vi "LDA+_An_Analysis_mode.vi"(6 "Second Graph":T2={"Plot 1"=1, "Plot 2"=2, "Save graph"=0, "Plot Type"=enum."Voltage trace"} {"Save graph" items=["Do not save plot", "Save plot"]; "Plot 2" items=["Nothing", "Prop 2 (U)"]; "Plot 1" items=["Nothing", "Prop 2 (U)"]}, 7 "Running Code?":bool, 9 "First Graph":T2={"Plot 1"=1, "Plot 2"=2, "Save graph"=0, "Plot Type"=enum."Voltage trace"} {"Save graph" items=["Do not save plot", "Save plot"]; "Plot 2" items=["Nothing", "Prop 2 (U)"]; "Plot 1" items=["Nothing", "Prop 2 (U)"]}) -> (0 "Second Graph out":T2={"Plot 1"=1, "Plot 2"=2, "Save graph"=0, "Plot Type"=enum."Voltage trace"} {"Save graph" items=["Do not save plot", "Save plot"]; "Plot 2" items=["Nothing", "Prop 2 (U)"]; "Plot 1" items=["Nothing", "Prop 2 (U)"]}, 3 "First Graph out":T2={"Plot 1"=1, "Plot 2"=2, "Save graph"=0, "Plot Type"=enum."Voltage trace"} {"Save graph" items=["Do not save plot", "Save plot"]; "Plot 2" items=["Nothing", "Prop 2 (U)"]; "Plot 1" items=["Nothing", "Prop 2 (U)"]})   [LabVIEW 2017]
uses:
  Controls/Graph_Type.ctl
  Globals/Meas_global.vi
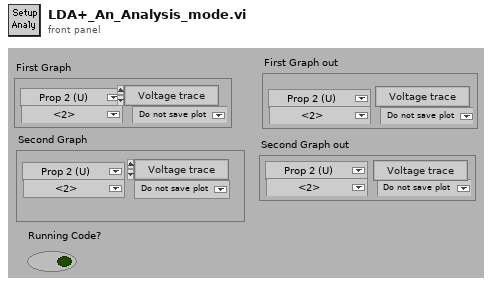
[diagram p1: front panel]
types:
  T1 = typedef "Graph_Type.ctl" = enum16{"Show no graph", "Voltage trace", "Velocity trace", "Vel histogram", "Spectrum", "f.E(f) v Log f", "Auto-Corr"}
  T2 = cluster{"Plot 1":u16, "Plot 2":u16, "Save graph":u16, "Plot Type":T1}
  T3 = typedef "Analysis_info_cluster.ctl" = cluster{"Colour":u32, "Inst type":T4, "Inst name":string, "Symbol":string, "Code name":string, "Extra Info":string, "Inst Array":T5, "Extra Titles":string[], "Extra Values":string[], "U":dbl, "u^2":dbl, "u^3":dbl, "u^4":dbl, "Skew_u":dbl, "Kurt_u":dbl, "Sd Error in Mean":dbl, "% u'/U":dbl, "X":dbl, "Y":dbl, "Z":dbl, "Timescale integral Estimate":dbl, "Sd Error in Variance":dbl, "Calib File":path, "Calib Constants":dbl[], "Output Position":bool, "Full Stats":bool, "Av Sampling Rate":dbl, "Av No of Samples":dbl, "Total Meas Time (s)":dbl, "ADAM Ch Name":string, "Max value":dbl, "Min value":dbl, "Req Sample Rate Hz":dbl, "Sync Delay Time (s)":dbl, "Ch No":i16, "Device ID":string, "Use Latest Calib":bool, "Port":string}
  T4 = typedef "Inst_type.ctl" = enum16{"Propeller anemometer", "Raw voltage", "Pressure Transducer", "Pitot-static tube", "Preston tube", "Hot wire", "Cross wire 1", "Cross wire 2", "Generic Linear", "Generic Polynomial", "Generic BackPoly", "Fast FID", "Thermocouple", "Cold wire", "Pulsed Wire", "LDA Vel", "LDA Tran time", "LDA Arr time", "Microphone"}
  T5 = typedef "Instrument_Array.ctl" = enum16{"PWA", "LDA", "Analogue"}
  T6 = enum16{"Show no graph", "Voltage trace", "Velocity trace", " Vel histogram", "Spectrum", "f.E(f) v Log f", "Auto-Corr"}
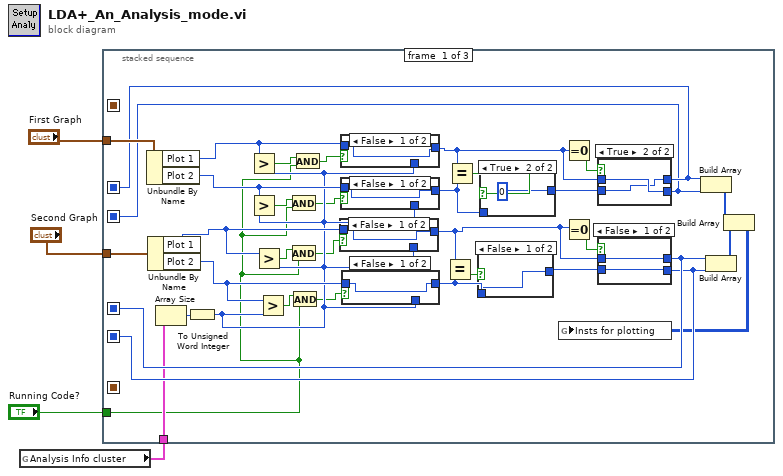
[diagram p0: block diagram]
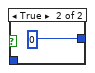
[diagram p9: hidden frame]
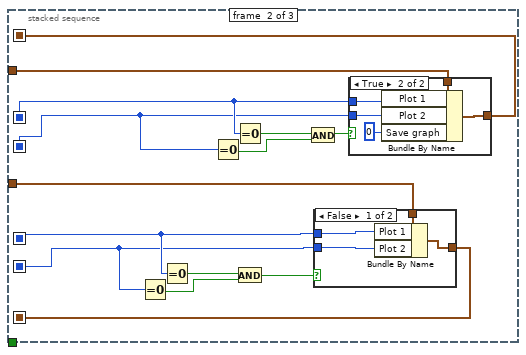
[diagram p10: hidden frame]
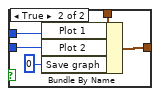
[diagram p11: hidden frame]
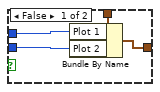
[diagram p12: hidden frame]
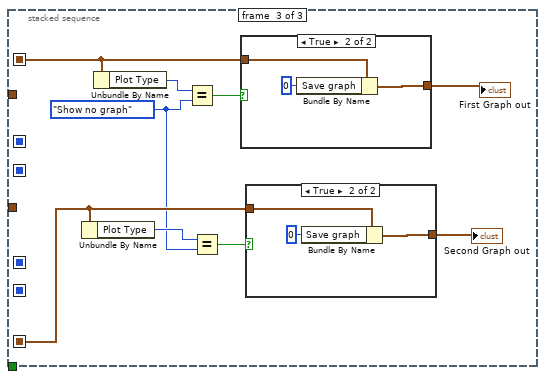
[diagram p13: hidden frame]
diagram:
  n1 = global read "Meas_global.vi" "Analysis Info cluster"() -> (w2:T3[])
  n2 = stacked-sequence {
    seq-local: [w25 _ _] -> [_ w70 _]
    seq-local: [w24 _ _] -> [_ w69 _]
    seq-local: [w20 _ _] -> [_ w64 _]
    seq-local: [w19 _ _] -> [_ w63 _]
    seq-local: [_ w60 _] -> [_ _ w98]
    seq-local: [_ w61 _] -> [_ _ w94]
    tunnel: "First Graph" -> [w34 w73 _]
    tunnel: "Second Graph" -> [w33 w67 _]
    tunnel: w2 -> [w14 _ _]
    tunnel: "Running Code?" -> [w6 _ _]
    frame #0 {
      n3 = Unbundle By Name(w34) -> ("Plot 1"=w32:u16, "Plot 2"=w31:u16)
      n4 = Unbundle By Name(w33) -> ("Plot 1"=w30:u16, "Plot 2"=w29:u16)
      n5 = Array Size(array=w14) -> (size(s)=w39:i32)
      n6 = To Unsigned Word Integer(number=w39) -> (unsigned 16bit integer=w15:u16)
      n7 = Greater?(x=w32, y=w15) -> (0:w12:bool)
      n8 = Greater?(x=w31, y=w15) -> (0:w11:bool)
      n9 = Greater?(x=w30, y=w15) -> (0:w8:bool)
      n10 = Greater?(x=w29, y=w15) -> (0:w9:bool)
      n11 = And(x=w11, y=w6) -> (x .and. y?=w5:bool)
      n12 = And(x=w8, y=w6) -> (x .and. y?=w10:bool)
      n13 = And(x=w9, y=w6) -> (x .and. y?=w7:bool)
      n14 = And(x=w12, y=w6) -> (x .and. y?=w13:bool)
      n15 = case shown="False" w10 {
        tunnel: [w54 w55] -> w22
        tunnel: w30 -> [w54 _]
        tunnel: w15 -> [_ w55]
        frame False {
        }
        frame True {
        }
      }
      n16 = case shown="False" w13 {
        tunnel: [w50 w51] -> w27
        tunnel: w32 -> [w50 _]
        tunnel: w15 -> [_ w51]
        frame False {
        }
        frame True {
        }
      }
      n17 = case shown="False" w5 {
        tunnel: [w52 w53] -> w36
        tunnel: w31 -> [w52 _]
        tunnel: w15 -> [_ w53]
        frame False {
        }
        frame True {
        }
      }
      n18 = case shown="False" w7 {
        tunnel: [w56 w57] -> w38
        tunnel: w29 -> [w56 _]
        tunnel: w15 -> [_ w57]
        frame False {
        }
        frame True {
        }
      }
      n19 = Equal?(x=w22, y=w38) -> (x = y?=w37:bool)
      n20 = Equal?(x=w27, y=w36) -> (x = y?=w35:bool)
      n21 = case shown="False" w37 {
        tunnel: [w58 u16 0] -> w21
        tunnel: w38 -> [w58 _]
        frame False {
        }
        frame True {
        }
      }
      n22 = case shown="True" w35 {
        tunnel: [w48 u16 0] -> w26
        tunnel: w36 -> [w48 _]
        frame False {
        }
        frame True {
        }
      }
      n23 = Equal To 0?(x=w27) -> (x = 0?=w28:bool)
      n24 = Equal To 0?(x=w22) -> (x = 0?=w23:bool)
      n25 = case shown="True" w28 {
        tunnel: [w44 w47] -> w24
        tunnel: w27 -> [w45 w47]
        tunnel: [w45 w46] -> w25
        tunnel: w26 -> [w44 w46]
        frame False {
        }
        frame True {
        }
      }
      n26 = case shown="False" w23 {
        tunnel: [w40 w43] -> w19
        tunnel: w22 -> [w41 w43]
        tunnel: [w41 w42] -> w20
        tunnel: w21 -> [w40 w42]
        frame False {
        }
        frame True {
        }
      }
      n27 = Build Array(w25, w24) -> (w18:u16[])
      n28 = Build Array(w20, w19) -> (w17:u16[])
      n29 = Build Array(w18, w17) -> (w16:u16[][])
      n30 = global write "Meas_global.vi" "Insts for plotting"(w16) -> ()
    }
    frame #1 {
      n31 = Equal To 0?(x=w63) -> (x = 0?=w66:bool)
      n32 = Equal To 0?(x=w64) -> (x = 0?=w65:bool)
      n33 = Equal To 0?(x=w69) -> (x = 0?=w71:bool)
      n34 = Equal To 0?(x=w70) -> (x = 0?=w72:bool)
      n35 = And(x=w65, y=w66) -> (x .and. y?=w62:bool)
      n36 = And(x=w72, y=w71) -> (x .and. y?=w68:bool)
      n37 = case shown="False" w62 {
        tunnel: [w77 w82] -> w61
        tunnel: w63 -> [w76 w81]
        tunnel: w64 -> [w75 w80]
        tunnel: w67 -> [w74 w79]
        frame False {
          n38 = Bundle By Name(cluster=w74, "Plot 1"=w75, "Plot 2"=w76) -> (w77:T2)
        }
        frame True {
          n39 = Bundle By Name(cluster=w79, "Plot 1"=w80, "Plot 2"=w81, "Save graph"=0) -> (w82:T2)
        }
      }
      n40 = case shown="True" w68 {
        tunnel: [w86 w91] -> w60
        tunnel: w69 -> [w85 w90]
        tunnel: w70 -> [w84 w89]
        tunnel: w73 -> [w83 w88]
        frame False {
          n41 = Bundle By Name(cluster=w83, "Plot 1"=w84, "Plot 2"=w85) -> (w86:T2)
        }
        frame True {
          n42 = Bundle By Name(cluster=w88, "Plot 1"=w89, "Plot 2"=w90, "Save graph"=0) -> (w91:T2)
        }
      }
    }
    frame #2 {
      w93 = T6."Show no graph" ("Plot Type")
      n43 = Unbundle By Name(w94) -> ("Plot Type"=w95:T1)
      n44 = Unbundle By Name(w98) -> ("Plot Type"=w100:T1)
      n45 = Equal?(x=w100, y=w93) -> (x = y?=w99:bool)
      n46 = Equal?(x=w95, y=w93) -> (x = y?=w96:bool)
      n47 = case shown="True" w99 {
        tunnel: w98 -> [w105 w108]
        tunnel: [w105 w106] -> w97
        frame False {
        }
        frame True {
          n48 = Bundle By Name(cluster=w108, "Save graph"=u16 0) -> (w106:T2)
        }
      }
      "First Graph out" <- w97
      n49 = case shown="True" w96 {
        tunnel: w94 -> [w101 w104]
        tunnel: [w101 w102] -> w92
        frame False {
        }
        frame True {
          n50 = Bundle By Name(cluster=w104, "Save graph"=u16 0) -> (w102:T2)
        }
      }
      "Second Graph out" <- w92
    }
  }
